vi "ex_11.vi"() -> ()   [LabVIEW 2020]
panel:
  out "Out 3":i32[][](array[numeric])
  out "Out 2":i32[][](array[numeric])
  out "Out 1":i32[][](array[numeric])
  in  "M":i32
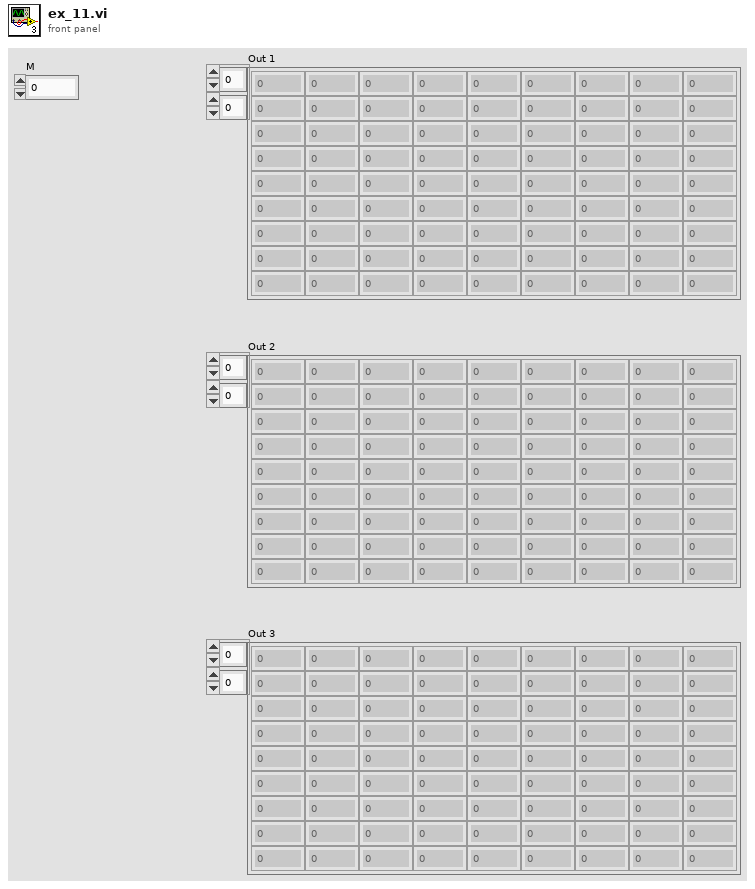
[diagram p1: front panel]
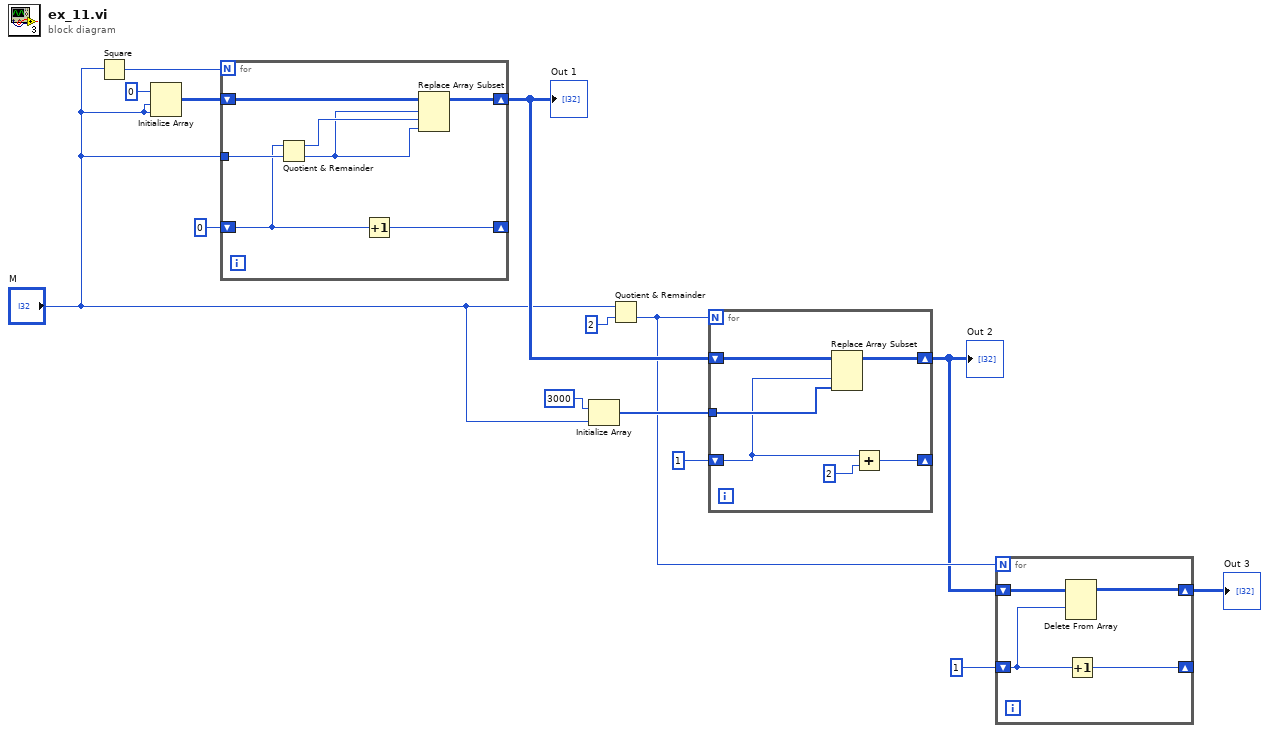
[diagram p0: block diagram]
diagram:
  n1 = Square(x="M") -> (x^2=w11:i32)
  n2 = Initialize Array(0, "M", "M") -> (w13:i32[][])
  n3 = for {
    N: w11 -> [_]
    shift-right: [w20] -> w9
    shift-left: w13 -> [w21]
    tunnel: "M" -> [w19]
    shift-right: [w18] -> _
    shift-left: 0 -> [w17]
    n4 = Quotient & Remainder(x=w17, y=w19) -> (x-y*floor(x/y)=w16:i32, floor(x/y)=w15:i32)
    n5 = Increment(x=w17) -> (x+1=w18:i32)
    n6 = Replace Array Subset(array=w21, new element=w15, index (row)=w15, index (col)=w16) -> (w20:i32[][])
  }
  "Out 1" <- w9
  n7 = Initialize Array(3000, "M") -> (w5:i32[])
  n8 = Quotient & Remainder(x="M", y=2) -> (floor(x/y)=w2:i32)  [unwired: 1 out]
  n9 = for {
    N: w2 -> [_]
    shift-right: [w27] -> _
    shift-left: 1 -> [w22]
    shift-right: [w24] -> w1
    shift-left: w9 -> [w25]
    tunnel: w5 -> [w23]
    n10 = Replace Array Subset(array=w25, new element=w23, index (col)=w22) -> (w24:i32[][])  [unwired: 1 in]
    n11 = Add(x=w22, y=2) -> (x+y=w27:i32)
  }
  "Out 2" <- w1
  n12 = for {
    N: w2 -> [_]
    shift-right: [w28] -> _
    shift-left: 1 -> [w29]
    shift-right: [w31] -> w3
    shift-left: w1 -> [w30]
    n13 = Delete From Array(array=w30, index (row)=w29) -> (array with subset deleted=w31:i32[][])  [unwired: 2 in, 1 out]
    n14 = Increment(x=w29) -> (x+1=w28:i32)
  }
  "Out 3" <- w3
